vi "State Actor Teardown.vi"(7 "Self Actor":refnum<class "Self Actor.lvclass">, 10 "Error":errorcluster, 11 "Destroying Self Actor State in":refnum<class "Destroying Self Actor State.lvclass">) -> (0 "error out":errorcluster, 2 "Teardown?":bool)   [LabVIEW 2021, in "LVCAM.lvlib" / "Destroying Self Actor State.lvclass"]
uses:
  Destroying Self Actor State.lvclass
  Self Actor/Self Actor.lvclass
  C:/PPLs/LabVIEW-Composed-Actor-Model-LVCAM/LabVIEW-Composed-Actor-Model-LVCAM/LVCAM/LVCAM/Actor/Actor.lvclass
  Msgs/Actor Destroy/Actor Destroy Msg Strategy/Actor Destroy Msg Strategy.lvclass
  C:/PPLs/LabVIEW-Composed-Actor-Model-LVCAM/LabVIEW-Composed-Actor-Model-LVCAM/LVCAM/LVCAM/Msg Strategy/Msg Strategy.lvclass
  Msgs/Actor Last Ack/Actor Last Ack Msg Strategy/Actor Last Ack Msg Strategy.lvclass
  Destroying Self Actor State.lvclass/Destroying Self Actor State.ctl
  Self Actor/Self Msg Send.vi
  Self Actor/Call Msg Send.vi
  C:/PPLs/LabVIEW-Composed-Actor-Model-LVCAM/LabVIEW-Composed-Actor-Model-LVCAM/LVCAM/Msgs/Actor Create/Actor Create/Actor Create.lvclass
  C:/PPLs/LabVIEW-Composed-Actor-Model-LVCAM/LabVIEW-Composed-Actor-Model-LVCAM/LVCAM/Msgs/Actor Destroy/Actor Destroy/Actor Destroy.lvclass
  C:/PPLs/LabVIEW-Composed-Actor-Model-LVCAM/LabVIEW-Composed-Actor-Model-LVCAM/LVCAM/Msgs/Actor Last Ack/Actor Last Ack/Actor Last Ack.lvclass
  C:/PPLs/LabVIEW-Composed-Actor-Model-LVCAM/LabVIEW-Composed-Actor-Model-LVCAM/LVCAM/LVCAM/Self Actor/Self Actor.lvclass
  C:/PPLs/LabVIEW-Composed-Actor-Model-LVCAM/LabVIEW-Composed-Actor-Model-LVCAM/LVCAM/Msgs/Actor Destroy/Actor Destroy Msg Strategy/Actor Destroy Msg Strategy.lvclass
  C:/PPLs/LabVIEW-Composed-Actor-Model-LVCAM/LabVIEW-Composed-Actor-Model-LVCAM/LVCAM/Msgs/Actor Last Ack/Actor Last Ack Msg Strategy/Actor Last Ack Msg Strategy.lvclass
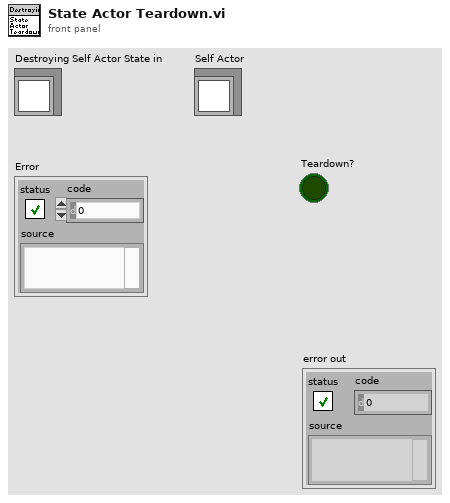
[diagram p1: front panel]
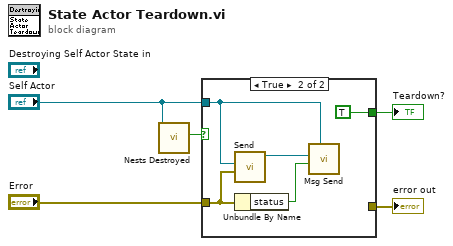
[diagram p0: block diagram]
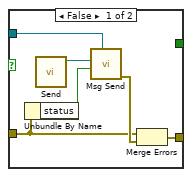
[diagram p2: hidden frame]
diagram:
  n1 = call "Nests Destroyed.vi"("Self Actor in"="Self Actor") -> ("Nests Destroyed?"=w1:bool)  [unwired: 9 in, 1 out]
  n2 = case shown="True" w1 {
    tunnel: "Self Actor" -> [w9 w14]
    tunnel: "Error" -> [w7 w13]
    tunnel: [_ TRUE ("Destroyed?")] -> w5
    tunnel: [w8 _] -> w2
    frame False {
      n3 = Unbundle By Name(w7) -> ("status"=w6:bool)
      n4 = call "Send.vi"() -> ("Actor Destroy Msg Strategy out"=w11:refnum<class "Actor Destroy Msg Strategy.lvclass">)  [unwired: 11 in]
      n5 = call-poly "Msg Send.vi"("Actor"=w9, "Priority Msg?"=w6, "Msg"=w11) -> ("error out"=w10:errorcluster)  [unwired: 8 in]
      n6 = Merge Errors(w7, w10) -> (w8:errorcluster)
    }
    frame True {
      n7 = call "Send.vi"("Nest Error"=w13, "Nest Actor"=w14) -> ("Actor Last Ack Msg Strategy out"=w15:refnum<class "Actor Last Ack Msg Strategy.lvclass">)  [unwired: 9 in]
      n8 = Unbundle By Name(w13) -> ("status"=w12:bool)
      n9 = call-poly "Msg Send.vi"("Actor"=w14, "Priority Msg?"=w12, "Msg"=w15) -> ()  [unwired: 8 in, 1 out]
    }
  }
  "error out" <- w2
  "Teardown?" <- w5
